vi "List Non-Volatile User Scripts.vi"(8 "error in":errorcluster, 11 "VISA resource name":refnum<visa-resource-name>) -> (0 "error out":errorcluster, 1 "Scripts":string[](array[string]), 3 "VISA resource name out":refnum<visa-resource-name>, 4 "Command String":string)   [LabVIEW 2012, in "Keithley 2600 Series.lvlib"]
doc: "This VI gets a list of user scripts that are currently in the instrument's non-volatile memory.\n\n<b>Functions and Attributes Used</b>\nscript.user.catalog()"
uses:
  Keithley 2600 Series.lvlib
panel:
  # "(c) 2008 Keithley Instruments, Inc.  ALL RIGHTS RESERVED."
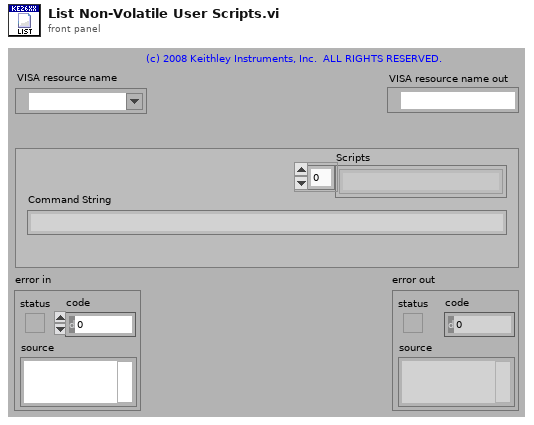
[diagram p1: front panel]
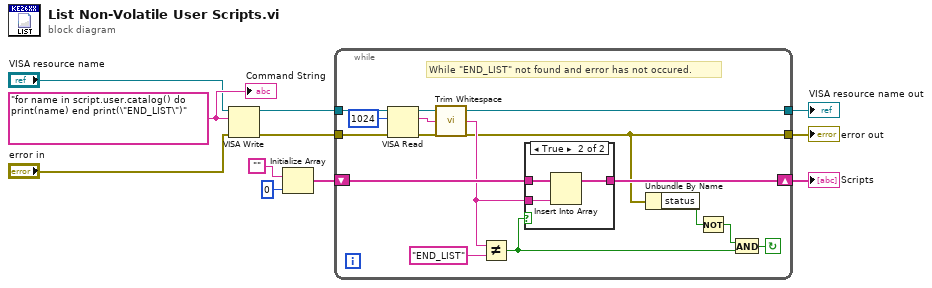
[diagram p0: block diagram]
diagram:
  w7 = "for name in script.user.catalog() do print(name) end print(\"END_LIST\")" ("write buffer")
  n1 = VISA Write(VISA resource name="VISA resource name", write buffer=w7, error in (no error)="error in") -> (VISA resource name out=w9:refnum<visa-resource-name>, error out=w5:errorcluster)  [unwired: 1 out]
  n2 = Initialize Array("", 0 ("dimension size")) -> (w2:string[])
  n3 = while {
    tunnel: w9 -> [w24]
    tunnel: w5 -> [w23]
    tunnel: [w16] -> w11
    tunnel: [w21] -> w8
    shift-right: [w19] -> w1
    shift-left: w2 -> [w20]
    stop <- w14 continue-if-true
    # "While \"END_LIST\" not found and error has not occured."
    n4 = VISA Read(VISA resource name=w24, byte count=u32 1024, error in (no error)=w23) -> (VISA resource name out=w21:refnum<visa-resource-name>, read buffer=w18:string, error out=w16:errorcluster)  [unwired: 1 out]
    n5 = call <vilib>:"Trim Whitespace.vi"("string"=w18) -> ("trimmed string"=w17:string)  [unwired: 1 in]
    n6 = Not Equal?(x=w17, y="END_LIST") -> (x != y?=w12:bool)
    n7 = case shown="True" w12 {
      tunnel: w17 -> [_ w29]
      tunnel: w20 -> [w26 w28]
      tunnel: [w26 w27] -> w19
      frame False {
      }
      frame True {
        n8 = Insert Into Array(array=w28, new element=w29) -> (w27:string[])  [unwired: 1 in]
      }
    }
    n9 = Unbundle By Name(w16) -> ("status"=w15:bool)
    n10 = Not(x=w15) -> (.not. x?=w13:bool)
    n11 = And(x=w13, y=w12) -> (x .and. y?=w14:bool)
  }
  "error out" <- w11
  "VISA resource name out" <- w8
  "Scripts" <- w1
  "Command String" <- w7
